vi "QT_AllVIs.vi"   [LabVIEW 2024]
panel:
  # "Just a Place holder for all the VIs\nSee the diagram\n\n\nCh. Salzmann @ 1994-2008\n\nbuild 2593\n\n\nNote that it is meant not to be executable"
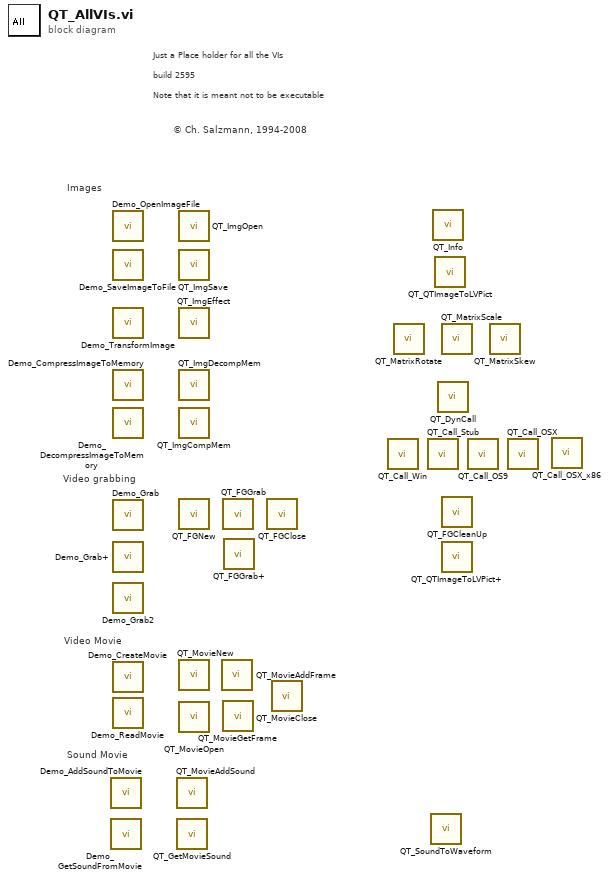
[diagram p0: block diagram]
diagram:
  # "Sound Movie"
  # "Video Movie"
  # "Video grabbing"
  # "Images"
  # "Just a Place holder for all the VIs\n\nbuild 2595\n\nNote that it is meant not to be executable"
  # "© Ch. Salzmann, 1994-2008"
  n1 = call <userlib>:"Demo_AddSoundToMovie.vi"() -> ()  [unwired: 12 in]
  n2 = call <userlib>:"Demo_GetSoundFromMovie.vi"() -> ()  [unwired: 12 in]
  n3 = call <userlib>:"Demo_OpenImageFile.vi"() -> ()  [unwired: 1 in]
  n4 = call <userlib>:"Demo_SaveImageToFile.vi"() -> ()  [unwired: 1 in]
  n5 = call <userlib>:"Demo_TransformImage.vi"() -> ()  [unwired: 1 in]
  n6 = call <userlib>:"Demo_CompressImageToMemory.vi"() -> ()  [unwired: 1 in]
  n7 = call <userlib>:"Demo_DecompressImageToMemory.vi"() -> ()  [unwired: 1 in]
  n8 = call <userlib>:"Demo_Grab.vi"() -> ()  [unwired: 1 in]
  n9 = call <userlib>:"Demo_Grab+.vi"() -> ()  [unwired: 1 in]
  n10 = call <userlib>:"Demo_Grab2.vi"() -> ()  [unwired: 1 in]
  n11 = call <userlib>:"Demo_CreateMovie.vi"() -> ()  [unwired: 1 in]
  n12 = call <userlib>:"Demo_ReadMovie.vi"() -> ()  [unwired: 1 in]
  n13 = call <userlib>:"QT_MovieAddSound.vi"() -> ()  [unwired: 18 in, 2 out]
  n14 = call <userlib>:"QT_GetMovieSound.vi"() -> ()  [unwired: 17 in, 3 out]
  n15 = call <userlib>:"QT_ImgOpen.vi"() -> ()  [unwired: 18 in, 2 out]
  n16 = call <userlib>:"QT_ImgSave.vi"() -> ()  [unwired: 19 in, 1 out]
  n17 = call <userlib>:"QT_ImgEffect.vi"() -> ()  [unwired: 18 in, 2 out]
  n18 = call <userlib>:"QT_ImgDecompMem.vi"() -> ()  [unwired: 17 in, 3 out]
  n19 = call <userlib>:"QT_ImgCompMem.vi"() -> ()  [unwired: 17 in, 3 out]
  n20 = call <userlib>:"QT_FGNew.vi"() -> ()  [unwired: 18 in, 2 out]
  n21 = call <userlib>:"QT_MovieNew.vi"() -> ()  [unwired: 18 in, 2 out]
  n22 = call <userlib>:"QT_MovieOpen.vi"() -> ()  [unwired: 17 in, 3 out]
  n23 = call <userlib>:"QT_MovieAddFrame.vi"() -> ()  [unwired: 18 in, 2 out]
  n24 = call <userlib>:"QT_FGGrab.vi"() -> ()  [unwired: 16 in, 4 out]
  n25 = call <userlib>:"QT_MovieGetFrame.vi"() -> ()  [unwired: 17 in, 3 out]
  n26 = call <userlib>:"QT_FGGrab+.vi"() -> ()  [unwired: 16 in, 4 out]
  n27 = call <userlib>:"QT_FGClose.vi"() -> ()  [unwired: 18 in, 2 out]
  n28 = call <userlib>:"QT_MovieClose.vi"() -> ()  [unwired: 18 in, 2 out]
  n29 = call <userlib>:"QT_Call_Win.vi"() -> ()  [unwired: 13 in, 7 out]
  n30 = call <userlib>:"QT_MatrixRotate.vi"() -> ()  [unwired: 13 in, 3 out]
  n31 = call <userlib>:"QT_Call_Stub.vi"() -> ()  [unwired: 13 in, 7 out]
  n32 = call <userlib>:"QT_SoundToWaveform.vi"() -> ()  [unwired: 10 in, 6 out]
  n33 = call <userlib>:"QT_Info.vi"() -> ()  [unwired: 13 in, 7 out]
  n34 = call <userlib>:"QT_QTImageToLVPict.vi"() -> ()  [unwired: 15 in, 5 out]
  n35 = call <userlib>:"QT_DynCall.vi"() -> ()  [unwired: 20 in, 8 out]
  n36 = call <userlib>:"QT_MatrixScale.vi"() -> ()  [unwired: 13 in, 3 out]
  n37 = call <userlib>:"QT_FGCleanUp.vi"() -> ()  [unwired: 19 in, 1 out]
  n38 = call <userlib>:"QT_QTImageToLVPict+.vi"() -> ()  [unwired: 12 in, 8 out]
  n39 = call <userlib>:"QT_Call_OS9.vi"() -> ()  [unwired: 13 in, 7 out]
  n40 = call <userlib>:"QT_MatrixSkew.vi"() -> ()  [unwired: 13 in, 3 out]
  n41 = call <userlib>:"QT_Call_OSX.vi"() -> ()  [unwired: 13 in, 7 out]
  n42 = call <userlib>:"QT_Call_OSX_x86.vi"() -> ()  [unwired: 13 in, 7 out]
